vi "get supported types.vi"(8 "error in":errorcluster, 11 "Scaling configuration in":refnum<class "Scaling configuration.lvclass">) -> (0 "error out":errorcluster, 2 "supported types":T1[](array[typedef]), 3 "Scaling configuration out":refnum<class "Scaling configuration.lvclass">)   [LabVIEW 2013, in "Scaling configuration.lvclass"]
doc: "Provides an interface for determining the targets supported by a given configuration/runtime class pairing. This should be overridden by any useful child class."
uses:
  Scaling configuration.lvclass
  <vilib>/NI/Tag Bus/tag/Data Type.ctl
  <vilib>/NI/Tag Bus/tag/tag descriptor.lvclass
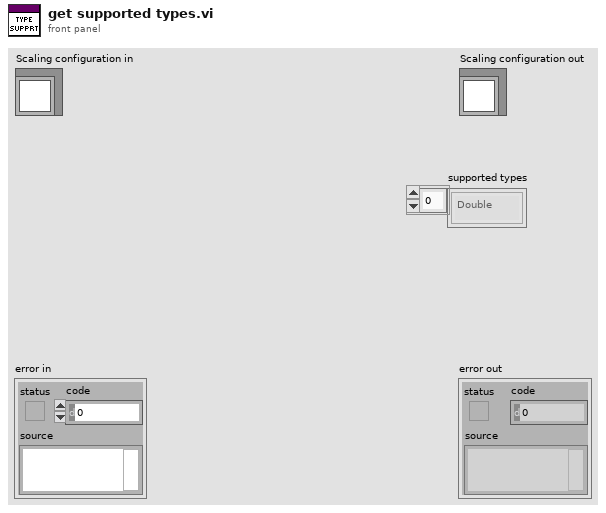
[diagram p1: front panel]
types:
  T1 = typedef "tag bus.lvlib/tag descriptor.lvclass/Data Type.ctl" = enum16{"Double", "Single", "I64", "I32", "I16", "I8", "U64", "U32", "U16", "U8", "Boolean", "String", "Array of Double", "Array of Single", "Array of I64", "Array of I32", "Array of I16", "Array of I8", "Array of U64", "Array of U32", "Array of U16", "Array of U8", "Array of Boolean", "Array of String"}
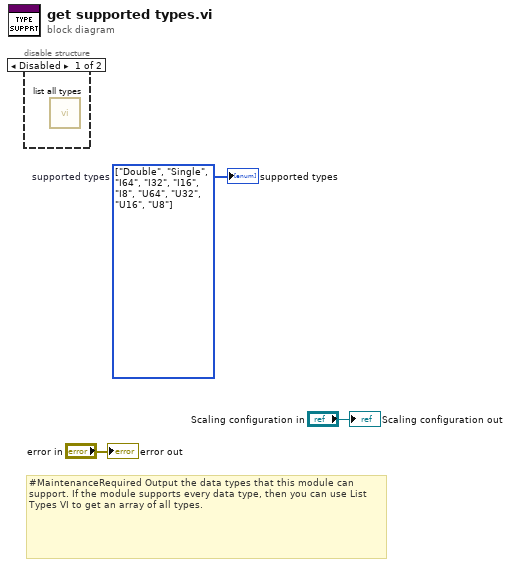
[diagram p0: block diagram]
diagram:
  w1 = T1[] [enum."Double", enum."Single", enum."I64", enum."I32", enum."I16", enum."I8", enum."U64", enum."U32", enum."U16", enum."U8"] items=["Double", "Single", "I64", "I32", "I16", "I8", "U64", "U32", "U16", "U8", "Boolean", "String", "Array of Double", "Array of Single", "Array of I64", "Array of I32", "Array of I16", "Array of I8", "Array of U64", "Array of U32", "Array of U16", "Array of U8", "Array of Boolean", "Array of String"]  # supported types
  # "#MaintenanceRequired Output the data types that this module can support. If the module supports every data type, then you can use List Types VI to get an array of all types."
  n1 = disable-structure shown="Disabled" {
    frame Disabled {
      n2 = call <vilib>:"list all types.vi"() -> ()  [unwired: 11 in, 1 out]
    }
    frame Enabled {
    }
  }
  "error out" <- "error in"
  "Scaling configuration out" <- "Scaling configuration in"
  "supported types" <- w1
